vi "Write configuration.vi"(8 "error in (no error)":errorcluster, 11 "AOTF in":refnum<class "AOTF.lvclass">) -> (0 "error out":errorcluster, 3 "AOTF out":refnum<class "AOTF.lvclass">)   [LabVIEW 2012]
doc: "Writes the configuration cluster into the configuration file. Configuration file is XML-based. It's name is <component ID>.xml"
uses:
  <vilib>/Distrio/Murmex/Murmex/Murmex.lvclass
  AOTF.lvclass
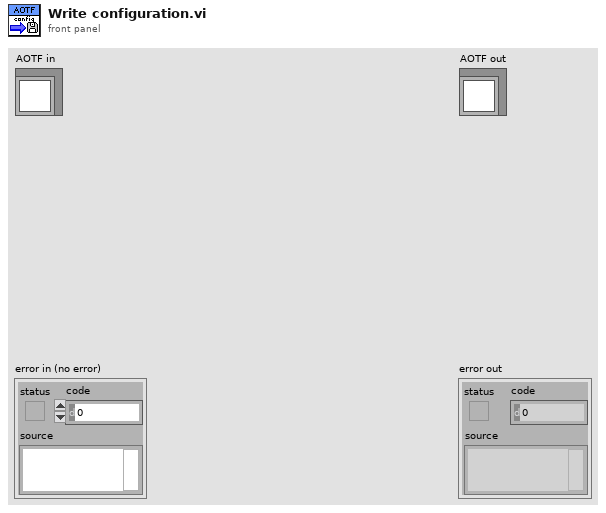
[diagram p1: front panel]
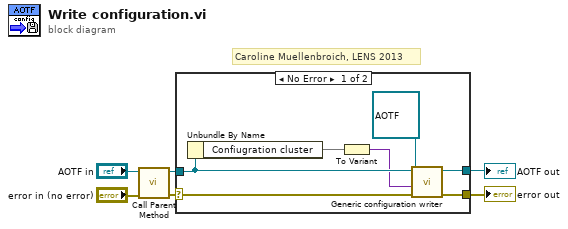
[diagram p0: block diagram]
diagram:
  # "Caroline Muellenbroich, LENS 2013"
  n1 = call-parent "Call Parent Method"("error in (no error)"="error in (no error)", "Murmex in"="AOTF in") -> ("error out"=w4:errorcluster, "Murmex out"=w3:refnum<class "AOTF.lvclass">)  [unwired: 8 in]
  n2 = case shown="No Error" w4 {
    selector: w4 -> [w11 w14]
    tunnel: [w12 w15] -> w2
    tunnel: w3 -> [w10 w15]
    tunnel: [w13 w14] -> w1
    frame No Error {
      n3 = Unbundle By Name(w10) -> ("Confiugration cluster"=w9)
      n4 = To Variant(anything=w9) -> (Variant=w8:variant)
      n5 = call <vilib>:"Generic configuration writer.vi"("error in (no error)"=w11, 9:w8, 10:refnum<class "AOTF.lvclass"> refnum ("AOTF"), "Murmex in"=w10) -> ("error out"=w13:errorcluster, "Murmex out"=w12:refnum<class "AOTF.lvclass">)  [unwired: 6 in]
    }
    frame Error {
    }
  }
  "error out" <- w1
  "AOTF out" <- w2
